vi "init_LM.vi"(7 "LM ID":T1=1 items=["none", "S1", "S2", "S3"], 8 "error in (no error)":errorcluster caption="错误输入（无错误）", 9 "CAN node ID":u32, 10 "device index":u32, 11 "LimitSwitch 输入":refnum<class "LimitSwitch.lvclass">) -> (0 "error out":errorcluster caption="错误输出", 3 "LimitSwitch 输出":refnum<class "LimitSwitch.lvclass">)   [LabVIEW 2016, in "MotionControl.lvlib" / "LimitSwitch.lvclass"]
uses:
  <userlib>/MotionControl/LimitSwitch/LimitSwitch.lvclass
  <userlib>/MotionControl/LimitSwitch/LM_ID.ctl
  <userlib>/MotionControl/LimitSwitch/LimitSwitch.lvclass/LimitSwitch.ctl
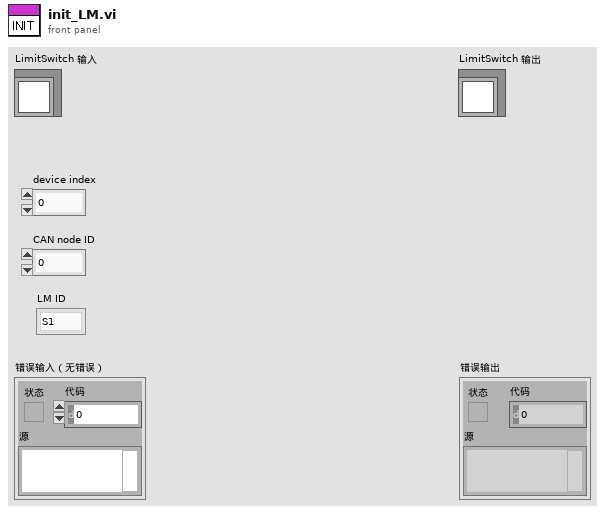
[diagram p1: front panel]
types:
  T1 = typedef "MotionControl.lvlib/LimitSwitch.lvclass/LM_ID.ctl" = i32
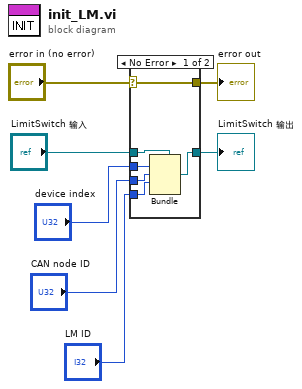
[diagram p0: block diagram]
diagram:
  n1 = case shown="No Error" "error in (no error)" {
    selector: "error in (no error)" -> [w13 w15]
    tunnel: [w13 w15] -> w6
    tunnel: [w9 w14] -> w4
    tunnel: "LimitSwitch 输入" -> [w12 w14]
    tunnel: "device index" -> [w11 _]
    tunnel: "CAN node ID" -> [w10 _]
    tunnel: "LM ID" -> [w8 _]
    frame No Error {
      n2 = Bundle(cluster=w12, w11, w10, w8) -> (w9:refnum<class "LimitSwitch.lvclass">)  [unwired: 2 in]
    }
    frame Error {
    }
  }
  "error out" <- w6
  "LimitSwitch 输出" <- w4
